vi "Teleop.vi"(9 "navX Device":T1={"Interface"={"Protocol"=enum."SPI", "Update Rate (4Hz-60Hz)"=50, "navX Open TypeDef"=variant(cluster{"DevStatus":errorcluster, "Handle":i32, "Controller":enum16{"Controller 1"}, "SPI Bus":enum16{"SPI On-Board, CS0", "SPI On-Board, CS1", "SPI On-Board, CS2", "SPI On-Board, CS3", "SPI MXP", "Invalid"}} {"DevStatus"={"status"=FALSE, "code"=0, "source"=""}, "Handle"=0, "Controller"=enum."Controller 1", "SPI Bus"=enum."SPI On-Board, CS0"})}, "Notify Packet"=refnum, "Loop VI Refnum"=refnum, "Ready to Close Occurrence Refnum"=refnum} {"Interface"."Update Rate (4Hz-60Hz)" min=4 max=60 step=1}, 10 "Match Info":T3={"Autonomous Elapsed Seconds"=0.0, "TeleOp Elapsed Seconds"=0.0, "Disabled Elapsed Seconds"=0.0, "Visited Autonomous"=FALSE, "Visited TeleOp"=FALSE, "Visited Disabled"=FALSE, "Autonomous Settings"={"Autonomous Style"=enum."Independent", "VI Refnum"=refnum}}, 11 "Call Context":T4) -> ()   [LabVIEW 2015]
doc: "This VI is called for each TeleOp packet received from the DS where the robot is not disabled. It is often used to read from the joysticks and update I/O or to update setpoints for timed control loops. It should complete and return within 20 milliseconds or it may miss DS packets."
uses:
  <vilib>/Rock Robotics/WPI/DriverStation/WPI_DriverStationDerivedRobotMode.ctl
  <vilib>/Rock Robotics/WPI/DriverStation/WPI_DriverStationMatch Info.ctl
  NavX Library/navX Library v2/TypeDefs/Z900_navX_DeviceTypeDef.ctl
  NavX Library/navX Library v2/TypeDefs/Z900_navX_ProtocolTypeDef.ctl
  NavX Library/navX Library v2/TypeDefs/Z900_navX_NotifyPacketTypeDef.ctl
  NavX Library/navX Library v2/TypeDefs/Z900_navX_ActionTypeDef.ctl
  <vilib>/Rock Robotics/Network Tables/SD Write Boolean.vi
  <vilib>/Rock Robotics/WPI/Utilities/WPI_GetSetVariantRefNum.vi
  Robot Global Data.vi
  NavX Library/navX Library v2/navX Library v2.lvlib
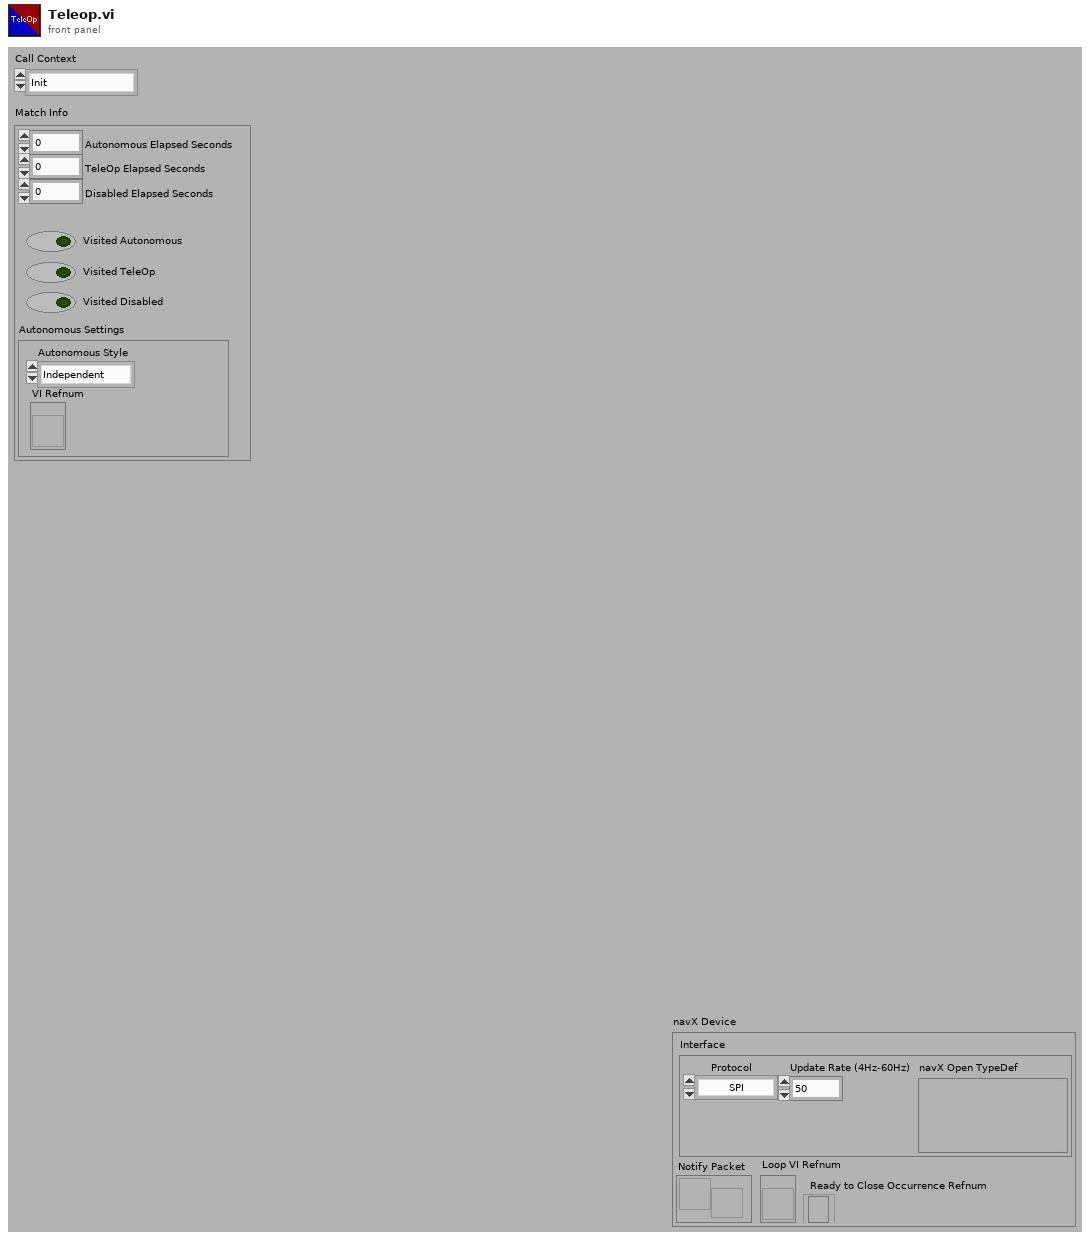
[diagram p1: front panel]
types:
  T1 = typedef "navX Library v2.lvlib/Z900_navX_DeviceTypeDef.ctl" = cluster{"Interface":cluster{"Protocol":T2, "Update Rate (4Hz-60Hz)":u8, "navX Open TypeDef":variant}, "Notify Packet":refnum<notifier>, "Loop VI Refnum":refnum<vi>, "Ready to Close Occurrence Refnum":refnum<k4>}
  T2 = typedef "navX Library v2.lvlib/Z900_navX_ProtocolTypeDef.ctl" = enum16{"SERIAL", "I2C", "SPI"}
  T3 = typedef "WPI_DriverStationMatch Info.ctl" = cluster{"Autonomous Elapsed Seconds":dbl, "TeleOp Elapsed Seconds":dbl, "Disabled Elapsed Seconds":dbl, "Visited Autonomous":bool, "Visited TeleOp":bool, "Visited Disabled":bool, "Autonomous Settings":cluster{"Autonomous Style":enum16{"Iterative", "Independent"}, "VI Refnum":refnum<vi>}}
  T4 = typedef "WPI_DriverStationDerivedRobotMode.ctl" = enum16{"Init", "Execute", "Stop"}
  T5 = typedef "navX Library v2.lvlib/Z900_navX_Flags_OpStatusTypeDef.ctl" = u8
  T6 = typedef "navX Library v2.lvlib/Z900_navX_Flags_CalibrationStatusTypeDef.ctl" = u8
  T7 = cluster{"Update Rate Hz":u8, "Accelerometer Full-Scale Range":u8, "Gyro Full-Scale Range":u16, "OP Status":T5, "Calibration Status":T6, "Sensor Status":cluster{"MOVING":bool, "YAW_STABLE":bool, "MAG_DISTURBANCE":bool, "ALTITUDE_VALID":bool, "SEALEVEL_PRESS_SET":bool, "FUSED_HEADING_VALID":bool}, "Self Test Status":cluster{"Gyro Passed":bool, "Accel Passed":bool, "Mag Passed":bool, "Baro Passed":bool, "Complete":bool}}
  T8 = typedef "WPI_RobotDriveDevRef.ctl" = cluster{"DevStatus":errorcluster, "Motors[]":T9[], "Square Inputs":bool, "Max Output":dbl}
  T9 = typedef "WPI_MotorControlDeviceRef.ctl" = cluster{"DeviceStatus":errorcluster, "Type":T10, "PWM":cluster{"PWM Channel":T11, "DeadBand":T12}, "CAN":cluster{"Device Number":u8, "Control Mode":T13, "Semaphore":T14, "Max Vout":dbl, "TalonSRX Control Mode":T15}, "Invert":bool}
  T10 = typedef "WPI_MotorControlType.ctl" = enum16{"PWM", "CAN", "CANTalonSRX"}
  T11 = typedef "FPGA_DIOPWMChannel.ctl" = enum8{"PWM 0", "PWM 1", "PWM 2", "PWM 3", "PWM 4", "PWM 5", "PWM 6", "PWM 7", "PWM 8", "PWM 9", "PWM MXP 0", "PWM MXP 1", "PWM MXP 2", "PWM MXP 3", "PWM MXP 4", "PWM MXP 5", "PWM MXP 6", "PWM MXP 7", "PWM MXP 8", "PWM MXP 9", "Invalid"}
  T12 = typedef "WPI_PWMDeadband.ctl" = cluster{"Name":string, "maxPositivePwm":i32, "minPositivePwm":i32, "centerPwm":i32, "maxNegativePwm":i32, "minNegativePwm":i32, "angularRange":u16}
  T13 = typedef "WPI_CANJaguar_ControlMode.ctl" = enum8{"Percent VBus", "Current", "Speed", "Position", "Voltage"}
  T14 = typedef "Semaphore RefNum" = refnum<k1>
  T15 = typedef "WPI_CANTalonSRX_APIControlMode.ctl" = enum8{"Percent VBus", "Speed", "Position", "Slave", "Unchanged / Invalid", "Voltage Compensation", "Current", "Motion Profile"}
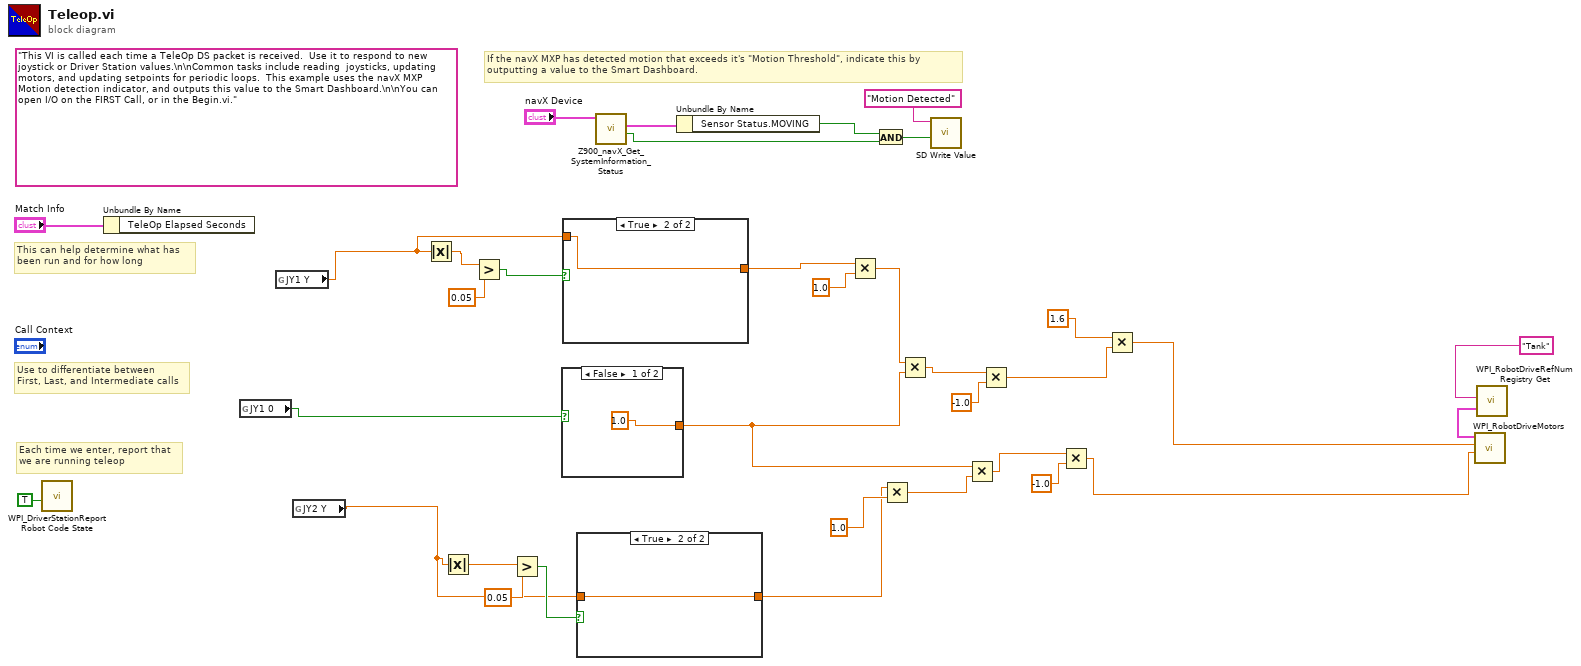
[diagram p0: block diagram]
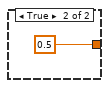
[diagram p2: hidden frame]
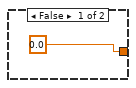
[diagram p3: hidden frame]
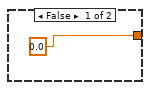
[diagram p4: hidden frame]
diagram:
  (unwired) "This VI is called each time a TeleOp DS packet is received.  Use it to respond to new joystick or Driver Station values.\n\nCommon tasks include reading  joysticks, updating motors, and updating setpoints for periodic loops.  This example uses the navX MXP Motion detection indicator, and outputs this value to the Smart Dashboard.\n\nYou can open I/O on the FIRST Call, or in the Begin.vi."
  # "If the navX MXP has detected motion that exceeds it's \"Motion Threshold\", indicate this by outputting a value to the Smart Dashboard."
  # "Each time we enter, report that\nwe are running teleop"
  # "Use to differentiate between\nFirst, Last, and Intermediate calls"
  # "This can help determine what has\nbeen run and for how long"
  n1 = call <vilib>:"WPI_DriverStationReport Robot Code State.vi"("TeleOp"=TRUE ("Autonomous")) -> ()  [unwired: 10 in, 1 out]
  n2 = Unbundle By Name("Match Info") -> ()  [unwired: 1 out]
  n3 = global read "Robot Global Data.vi" "JY1 0"() -> (w1:bool)
  n4 = global read "Robot Global Data.vi" "JY1 Y"() -> (w3:dbl)
  n5 = global read "Robot Global Data.vi" "JY2 Y"() -> (w2:dbl)
  n6 = Absolute Value(x=w3) -> (abs(x)=w8:dbl)
  n7 = Absolute Value(x=w2) -> (abs(x)=w7:dbl)
  n8 = Greater?(x=w8, y=0.05) -> (0:w26:bool)
  n9 = Greater?(x=w7, y=0.05) -> (0:w24:bool)
  n10 = case shown="False" w1 {
    tunnel: [1.0 0.5] -> w15
    frame False {
    }
    frame True {
    }
  }
  n11 = case shown="True" w26 {
    tunnel: [0.0 w38] -> w20
    tunnel: w3 -> [_ w38]
    frame False {
    }
    frame True {
    }
  }
  n12 = case shown="True" w24 {
    tunnel: [0.0 w40] -> w19
    tunnel: w2 -> [_ _]
    tunnel: w2 -> [_ w40]
    frame False {
    }
    frame True {
    }
  }
  n13 = call "Z900_navX_Get_SystemInformation_Status.vi"("navX Device"="navX Device") -> ("Connected"=w28:bool, "Status"=w30:T7)  [unwired: 7 in, 2 out]
  n14 = Unbundle By Name(w30) -> ("Sensor Status.MOVING"=w29:bool)
  n15 = Multiply(x=w20, y=1.0) -> (x*y=w16:dbl)
  n16 = And(x=w29, y=w28) -> (x .and. y?=w27:bool)
  n17 = Multiply(x=w19, y=1.0) -> (x*y=w14:dbl)
  n18 = Multiply(x=w16, y=w15) -> (x*y=w13:dbl)
  n19 = call-poly <vilib>:"SD Write Value.vi"("Boolean"=w27, "Name"="Motion Detected") -> ()  [unwired: 8 in, 2 out]
  n20 = Multiply(x=w15, y=w14) -> (x*y=w9:dbl)
  n21 = Multiply(x=w13, y=-1.0) -> (x*y=w5:dbl)
  n22 = Multiply(x=w9, y=-1.0) -> (x*y=w10:dbl)
  n23 = Multiply(x=1.6, y=w5) -> (x*y=w4:dbl)
  n24 = call <vilib>:"WPI_RobotDriveRefNum Registry Get.vi"("refnum name"="Tank") -> ("RobotDriveDevRef"=w17:T8)  [unwired: 1 in, 9 out]
  n25 = call <vilib>:"WPI_RobotDriveMotors.vi"("RightSpeed"=w10, "LeftSpeed"=w4, "RobotDriveDevRef"=w17) -> ()  [unwired: 6 in, 3 out]
